vi "_TEMPLATE.vi"(8 "error in (no error)":errorcluster) -> (0 "error out":errorcluster, 3 "Result":i32)   [LabVIEW 2018, in "Fujifilm X Series GFX System Digital Camera.lvlib"]
doc: "Terminates the software connection to the instrument."
uses:
  <instrlib>/Fujifilm X Series GFX System Digital Camera/Fujifilm X Series GFX System Digital Camera.lvlib
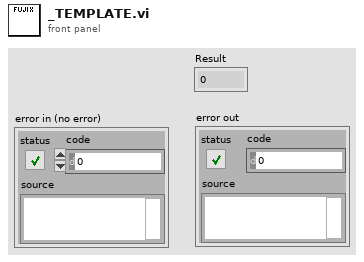
[diagram p1: front panel]
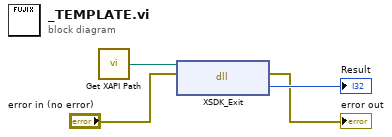
[diagram p0: block diagram]
diagram:
  n1 = call <instrlib>:"Get XAPI Path.vi"() -> ("XAPI Library Path"=w4:path)  [unwired: 1 in]
  n2 = dll-call lib="E:/fuji/SDK13100/REDISTRIBUTABLES/Windows/32bit/XAPI.dll" fn="XSDK_Exit"(path in=w4, error in="error in (no error)") -> (error out=→"error out":errorcluster, "result"=→"Result":i32)  [unwired: 1 in, 1 out]
